vi "Gas_Release_Control.vi"(5 "Extra Commands":string, 6 "Density Ratio":string="Carrier 1 only", 7 "Strength (% by volume)":dbl format="%.3f", 8 "Stack flowrate (l/min)":dbl format="%.2f", 9 "Source Status":T2) -> (0 "error out":errorcluster, 1 "Flowrates (kg/min)":dbl[](array[numeric]) format="%.2f", 2 "Source Est Time (s)":dbl, 3 "Flowrates Achieved?":bool)   [LabVIEW 2013]
uses:
  ADAM Controls/Client_Source_Status.ctl
  ADAM Controls/Client_Source.ctl
  ADAM Controls/Channel_names.ctl
  ADAM Controls/Module_type_ADAM.ctl
  ADAM Controls/Calib_type_ADAM.ctl
  ADAM Controls/Channel_State.ctl
  ADAM Controls/Ch_description_ADAM.ctl
  ADAM Controls/Function_ADAM.ctl
  ADAM Controls/Address.ctl
  ADAM Controls/Update_scan_value.ctl
  Anemometry/Anemometry Sub Vis/Controls/In_Range.ctl
  Anemometry/Anemometry Sub Vis/Globals/Preference_global.vi
  Anemometry/Anemometry Sub Vis/Globals/Extra_Commands_Global.vi
panel:
  out "Error String":string
  out "Currently on":T1=enum."Get Source Clients"
  out "Status of other Clients":string[](array[string])
  out "Source already correct?":bool
  out "No Other Clients are Using Source?":bool
  out "Source Clients":string[](array[string])
  # "-Carrier 1 only\n-Carrier 2 only\n-Enter Ratio"
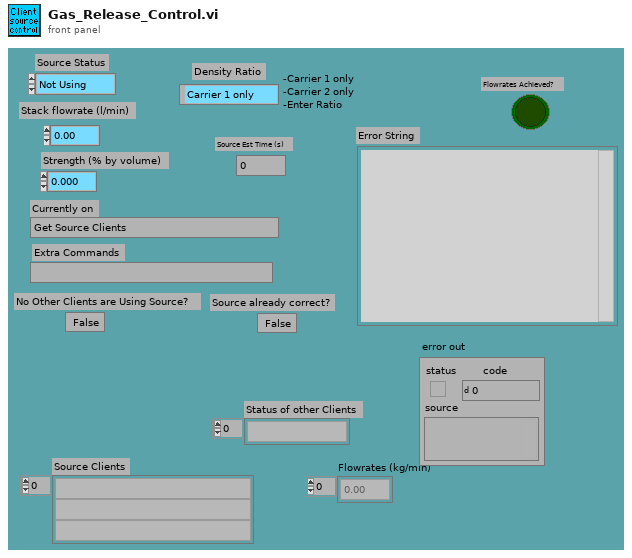
[diagram p1: front panel]
types:
  T1 = typedef "Client_Source.ctl" = enum16{"Start", "Get Source Clients", "Has this client liberty to control the source?", "Declare not using, other client already waiting", "Is the Source already correct?", "Declare waiting, other client is still using", "Control Hi-Tec", "Were the Hi-tecs able to achieve the flowrates?", "Declare source status", "Wait for source to Establish"}
  T2 = typedef "Client_Source_Status.ctl" = enum16{"Not Using", "Using", "Must Have"}
  T3 = typedef "Channel_names.ctl" = enum16{"Active Only", "Active + Off", "All Channels"}
  T4 = typedef "Ch_description_ADAM.ctl" = cluster{"Ch Name":string, "Type":T5, "Function":T6, "Ch State":T7, "Calibration type":T8, "A":dbl, "B":dbl, "C":dbl, "D":dbl, "Comments":string, "Address":T9, "String":string, "Duty":u16}
  T5 = typedef "Module_type_ADAM.ctl" = string
  T6 = typedef "Function_ADAM.ctl" = enum16{"Analogue Input", "Digital Input", "Event counter", "Event rate", "Analogue Output", "Digital Output", "Relay Output"}
  T7 = typedef "Channel_State.ctl" = enum16{"On", "Off", "Always On", "Always Off"}
  T8 = typedef "Calib_type_ADAM.ctl" = enum16{"Raw", "Bx + A", "Cx^2 + Bx + A", "Dx^3 + Cx^2 + Bx + A", "In Band", "Hi-Tec Q", "Hi-Tec M_dot", "Text"}
  T9 = typedef "Address.ctl" = cluster{"Main":i32, "Ch.":i32, "Sub":i32, "Port Name":string}
  T10 = typedef "Update_scan_value.ctl" = cluster{"Channel Name":string, "New Value":dbl}
  T11 = typedef "In_Range.ctl" = enum16{"%", "±", "% & ±"}
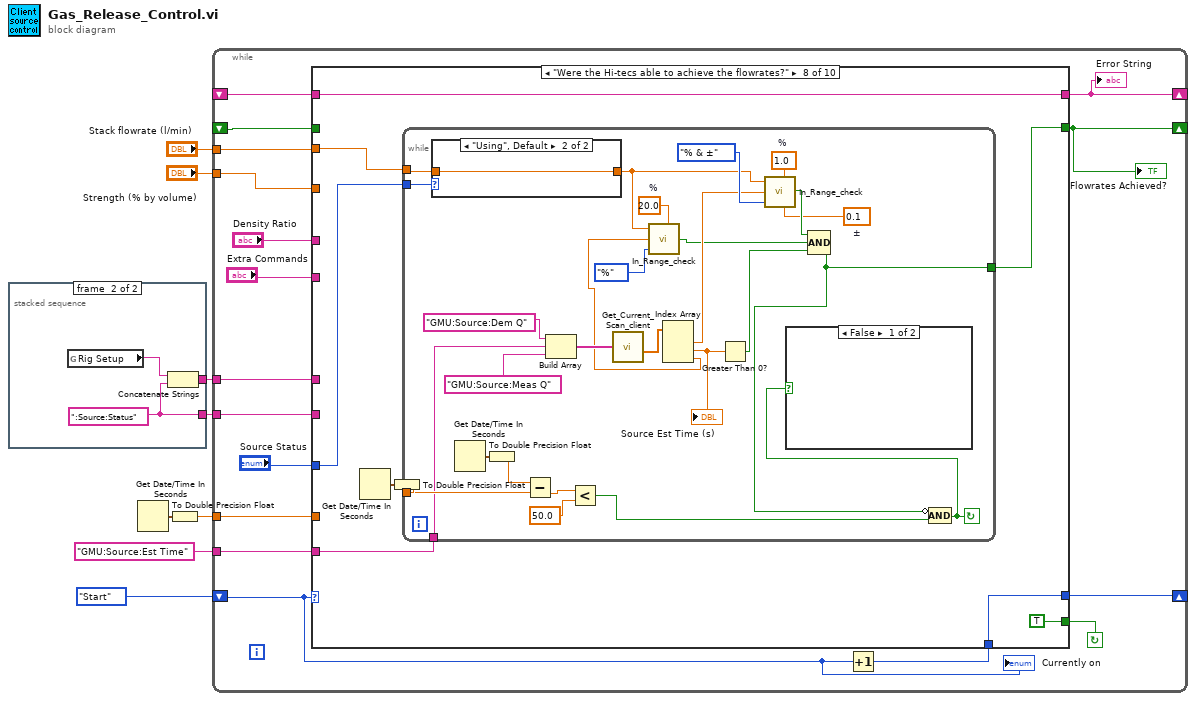
[diagram p0: block diagram]
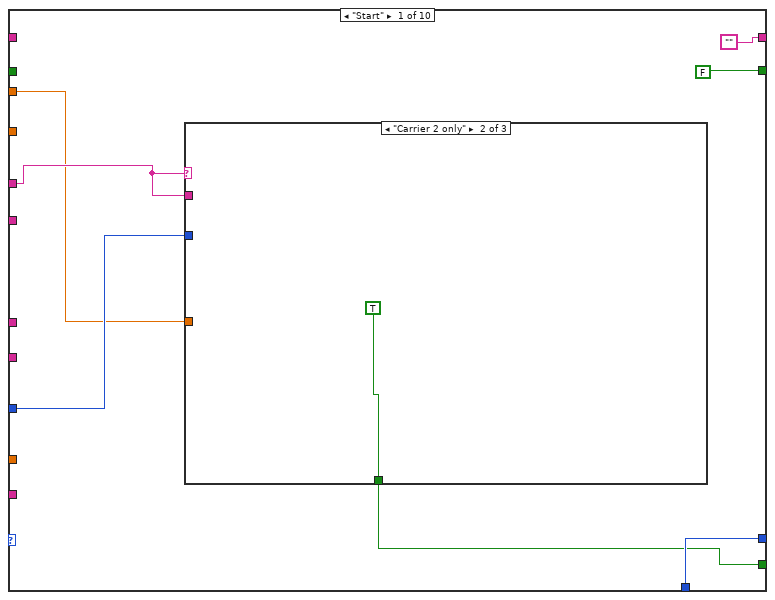
[diagram p2: hidden frame]
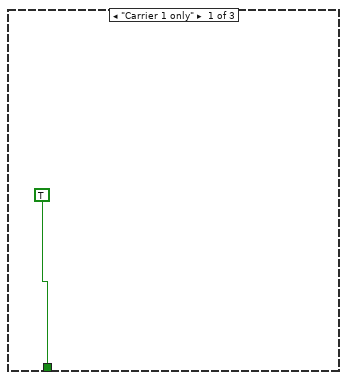
[diagram p3: hidden frame]
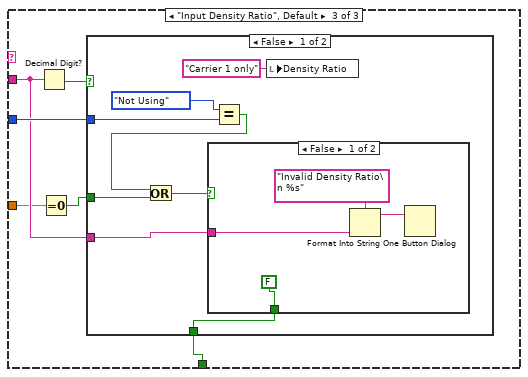
[diagram p4: hidden frame]
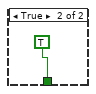
[diagram p5: hidden frame]
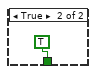
[diagram p6: hidden frame]
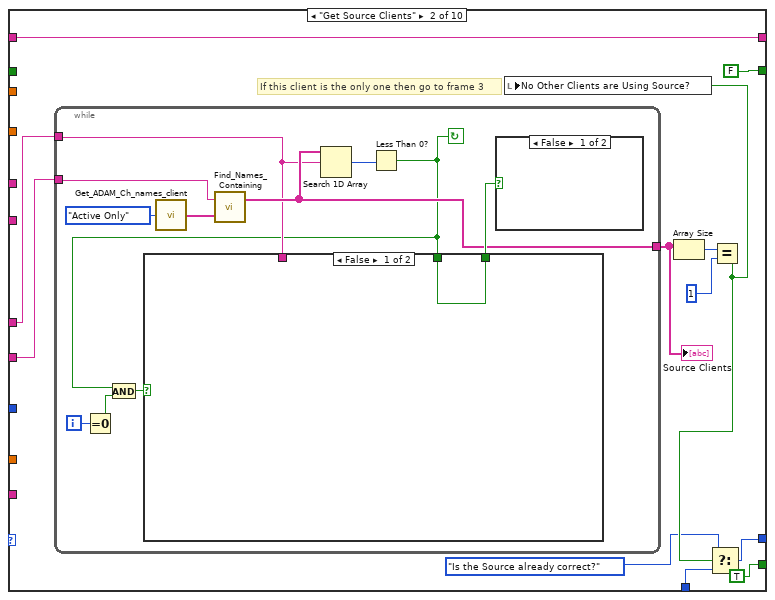
[diagram p7: hidden frame]
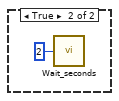
[diagram p8: hidden frame]
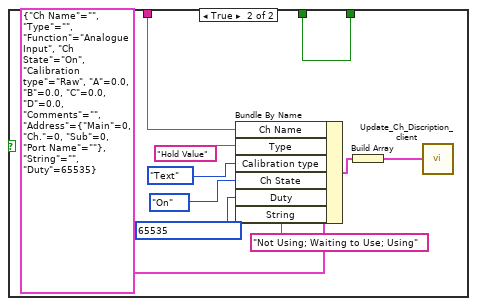
[diagram p9: hidden frame]
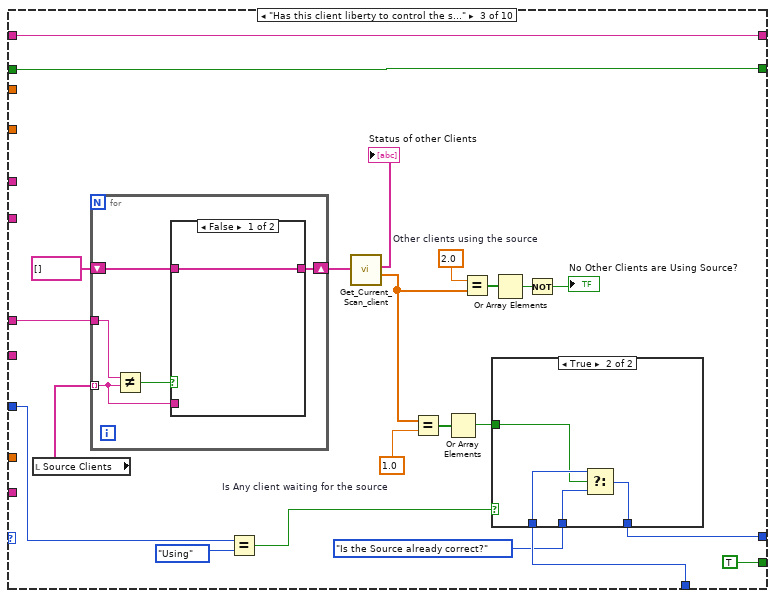
[diagram p10: hidden frame]
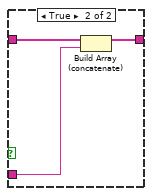
[diagram p12: hidden frame]
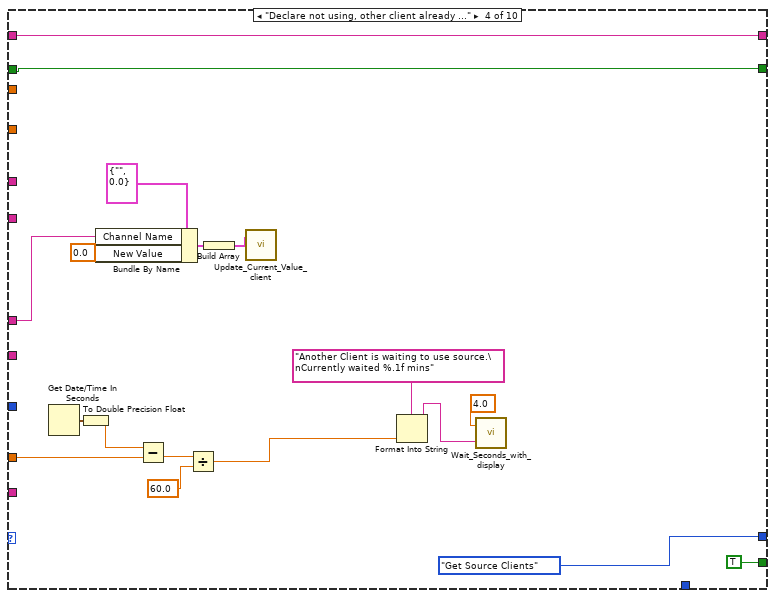
[diagram p13: hidden frame]
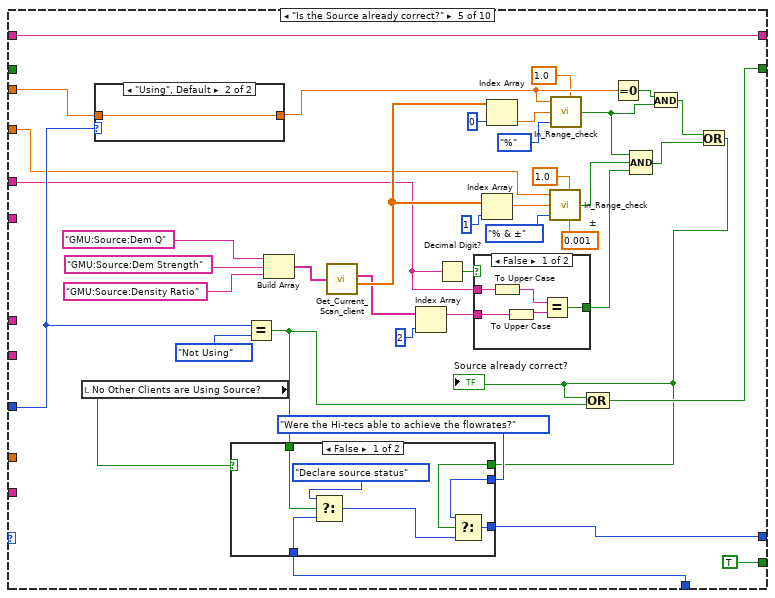
[diagram p14: hidden frame]
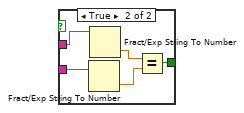
[diagram p15: hidden frame]
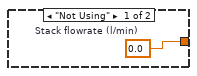
[diagram p16: hidden frame]
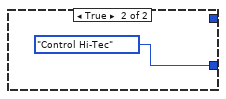
[diagram p17: hidden frame]
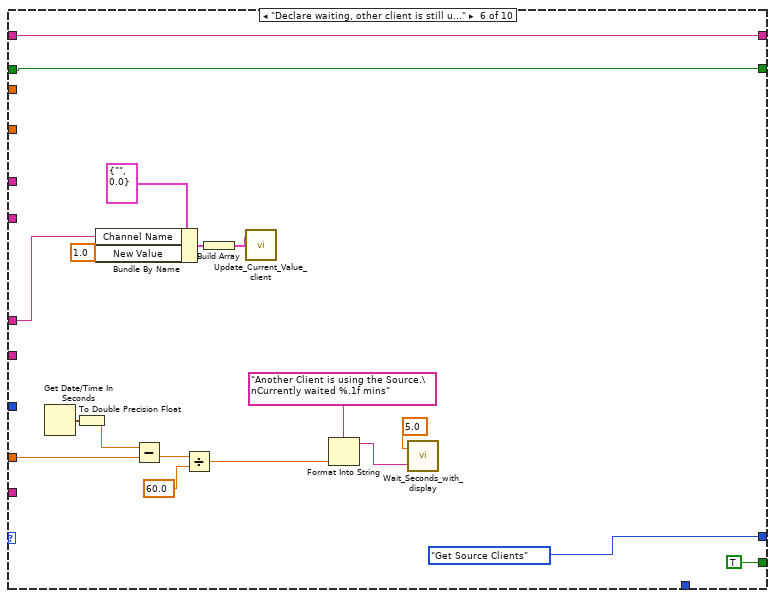
[diagram p18: hidden frame]
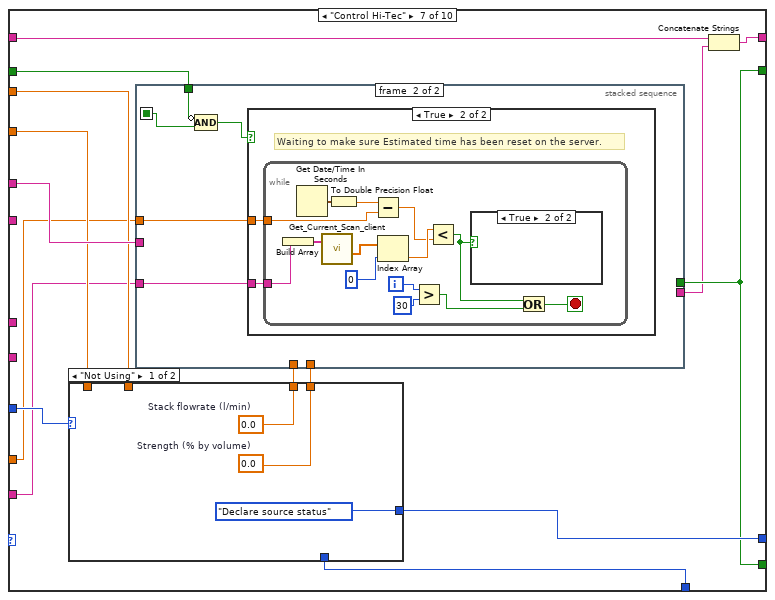
[diagram p19: hidden frame]
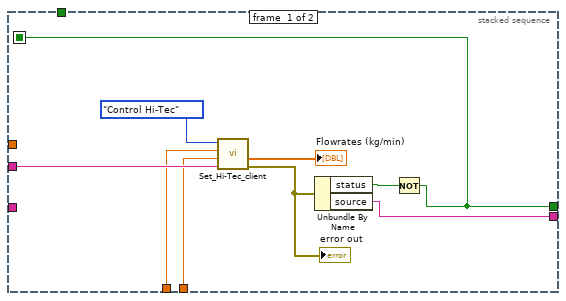
[diagram p20: hidden frame]
diagram:
  n1 = stacked-sequence {
    tunnel: [_ w11] -> w8
    tunnel: [_ w10] -> w7
    frame #0 {
      n2 = call "Run_EnFlo_Hub.vi"() -> ()  [unwired: 8 out]
    }
    frame #1 {
      w11 = ":Source:Status"
      n3 = global read "Preference_global.vi" "Rig Setup"() -> (w9:string)
      n4 = Concatenate Strings(w9, w11) -> (w10:string)
    }
  }
  n5 = Get Date/Time In Seconds() -> (seconds since 1Jan1904=w2:timestamp)
  n6 = To Double Precision Float(number=w2) -> (double precision float=w6:dbl)
  n7 = while {
    tunnel: w6 -> [w24]
    tunnel: w7 -> [w27]
    shift-left: Client_Source."Start" -> [w22]
    shift-right: [w23] -> _
    tunnel: w8 -> [w28]
    tunnel: "Stack flowrate (l/min)" -> [w18]
    tunnel: "Strength (% by volume)" -> [w17]
    shift-right: [w15] -> _
    shift-left: _ -> [w16]
    tunnel: "GMU:Source:Est Time" -> [w14]
    shift-right: [w12] -> _
    shift-left: _ -> [w13]
    stop <- w26 continue-if-true
    n8 = Increment(x=w22) -> (x+1=w25:T1)
    n9 = case shown="\"Were the Hi-tecs able to achieve the flowrates?\"" w22 {
      tunnel: w18 -> [w30 _ _ _ w178 _ w235 w281 _ w339]
      tunnel: w17 -> [_ _ _ _ w161 _ w233 _ _ _]
      tunnel: "Density Ratio" -> [w34 _ _ _ w153 _ w238 _ _ _]
      tunnel: w28 -> [_ w69 _ _ _ _ _ _ _ _]
      tunnel: [w35 w65 w107 Client_Source."Get Source Clients" w149 Client_Source."Get Source Clients" w232 w282 w323 w345] -> w23
      tunnel: w27 -> [_ w68 w114 w141 _ w218 _ _ w325 _]
      tunnel: [w33 TRUE TRUE TRUE TRUE TRUE w228 TRUE w317 FALSE] -> w26
      tunnel: w25 -> [w35 w64 w109 _ w179 _ w231 w282 w323 w345]
      tunnel: w24 -> [_ _ _ w139 _ w213 w229 _ _ _]
      tunnel: "Source Status" -> [w32 _ w98 _ w170 _ w237 w280 w324 w344]
      tunnel: "Extra Commands" -> [_ _ _ _ _ _ _ _ _ w342]
      tunnel: [FALSE FALSE w94 w131 w151 w208 w228 w279 w318 w340] -> w15
      tunnel: w16 -> [_ _ w94 w131 _ w208 w227 _ w318 w340]
      tunnel: w14 -> [_ _ _ _ _ _ w230 w277 _ _]
      tunnel: w13 -> [_ w58 w93 w129 w147 w206 w225 w276 w316 w338]
      tunnel: ["" w58 w93 w129 w147 w206 w226 w276 w315 w338] -> w12
      frame "Start" {
        n10 = case shown="\"Carrier 2 only\"" w34 {
          tunnel: w34 -> [_ _ w40]
          tunnel: [TRUE TRUE w41] -> w33
          tunnel: w32 -> [_ _ w42]
          tunnel: w30 -> [_ _ w39]
          frame "Carrier 1 only" {
            (unwired) TRUE
            (unwired) 0.0 ("Qc2")
          }
          frame "Carrier 2 only" {
            (unwired) TRUE
            (unwired) 0.0 ("Qc1")
          }
          frame "Input Density Ratio", Default {
            n11 = Decimal Digit?(1:w40) -> (0:w43:bool)
            n12 = Equal To 0?(x=w39) -> (x = 0?=w38:bool)
            n13 = case shown="False" w43 {
              tunnel: w42 -> [w50 _]
              tunnel: [w49 TRUE] -> w41
              tunnel: w40 -> [w48 _]
              tunnel: w38 -> [w45 _]
              frame False {
                n14 = Equal?(x=Client_Source_Status."Not Using" ("Source Status"), y=w50) -> (x = y?=w46:bool)
                n15 = Or(x=w46, y=w45) -> (x .or. y?=w44:bool)
                n16 = case shown="False" w44 {
                  tunnel: [FALSE TRUE] -> w49
                  tunnel: w48 -> [w55 _]
                  frame False {
                    n17 = Format Into String(format string="Invalid Density Ratio\n %s", w55) -> (resulting string=w53:string)  [unwired: 2 in, 1 out]
                    n18 = One Button Dialog(message=w53) -> ()  [unwired: 2 out]
                  }
                  frame True {
                  }
                }
                n19 = local write "Density Ratio"("Carrier 1 only" ("Density Ratio")) -> ()
              }
              frame True {
              }
            }
          }
        }
      }
      frame "Get Source Clients" {
        # "If this client is the only one then go to frame 3"
        n20 = while {
          tunnel: [w73] -> w62
          tunnel: w68 -> [w72]
          tunnel: w69 -> [w80]
          i -> [w77]
          stop <- w70 continue-if-true
          n21 = Equal To 0?(x=w77) -> (x = 0?=w76:bool)
          n22 = call "Get_ADAM_Ch_names_client.vi"("Channel names set"=Channel_names."Active Only") -> ("Ch names"=w78:string[])
          n23 = call "Find_Names_Containing.vi"("Ch names"=w78, "String to match"=w80) -> ("Matched Names"=w73:string[])  [unwired: 1 out]
          n24 = Search 1D Array(1D array=w73, element=w72) -> (index of element=w71:i32)  [unwired: 1 out]
          n25 = Less Than 0?(x=w71) -> (x < 0?=w70:bool)
          n26 = And(x=w70, y=w76) -> (x .and. y?=w75:bool)
          n27 = case shown="False" w75 {
            tunnel: w72 -> [_ w89]
            tunnel: [w82 w85] -> w74
            tunnel: w70 -> [w82 w85]
            frame False {
            }
            frame True {
              n28 = Bundle By Name(cluster=T4 {"Ch Name"="", "Type"="", "Function"=enum."Analogue Input", "Ch State"=enum."On", "Calibration type"=enum."Raw", "A"=0.0, "B"=0.0, "C"=0.0, "D"=0.0, "Comments"="", "Address"={"Main"=0, "Ch."=0, "Sub"=0, "Port Name"=""}, "String"="", "Duty"=65535} ("Ch Discription"), "Ch Name"=w89, "Type"=T5 "Hold Value", "Calibration type"=Calib_type_ADAM."Text", "Ch State"=Channel_State."On", "Duty"=u16 65535 ("Bundle Element"), "String"="Not Using; Waiting to Use; Using") -> (w87:T4)
              n29 = Build Array(w87) -> (w86:T4[])
              n30 = call "Update_Ch_Discription_client.vi"("Channels to update In"=w86) -> ()  [unwired: 1 out]
            }
          }
          n31 = case shown="False" w74 {
            frame False {
            }
            frame True {
              n32 = call "Wait_seconds.vi"("Seconds to wait"=u32 2) -> ()
            }
          }
        }
        "Source Clients" <- w62
        n33 = Array Size(array=w62) -> (size(s)=w67:i32)
        n34 = Equal?(x=w67, y=1) -> (x = y?=w61:bool)
        n35 = local write "No Other Clients are Using Source?"(w61) -> ()
        n36 = Select(t=Client_Source."Is the Source already correct?", s=w61, f=w64) -> (s? t:f=w65:T1)
      }
      frame "Has this client liberty to control the source?" {
        w106 = 2.0  # Other clients using the source
        w112 = 1.0  # Is Any client waiting for the source
        n37 = local read "Source Clients"() -> (w108:string[])
        n38 = for {
          tunnel: w108 -> [w120] mode=indexing
          tunnel: w114 -> [w124]
          shift-right: [w121] -> w104
          shift-left: string[] [] -> [w122]
          n39 = Not Equal?(x=w124, y=w120) -> (x != y?=w123:bool)
          n40 = case shown="False" w123 {
            tunnel: w122 -> [w125 w128]
            tunnel: [w125 w127] -> w121
            tunnel: w120 -> [_ w126]
            frame False {
            }
            frame True {
              n41 = Build Array (concatenate)(w128, w126) -> (w127:string[])
            }
          }
        }
        n42 = Equal?(x=w98, y=Client_Source_Status."Using" ("Source Status")) -> (x = y?=w97:bool)
        n43 = call "Get_Current_Scan_client.vi"("ADAM Ch Names"=w104) -> ("String values"=→"Status of other Clients":string[], "Numerical Values"=w101:dbl[])  [unwired: 2 out]
        n44 = Equal?(x=w101, y=w112) -> (x = y?=w111:bool[])
        n45 = Or Array Elements(Boolean array=w111) -> (logical OR=w102:bool)
        n46 = Equal?(x=w106, y=w101) -> (x = y?=w105:bool[])
        n47 = case shown="True" w97 {
          tunnel: w109 -> [_ w119]
          tunnel: [w115 w118] -> w107
          tunnel: w102 -> [_ w117]
          tunnel: Client_Source."Is the Source already correct?" -> [w115 w116]
          frame False {
          }
          frame True {
            n48 = Select(t=w119, s=w117, f=w116) -> (s? t:f=w118:T1)
          }
        }
        n49 = Or Array Elements(Boolean array=w105) -> (logical OR=w100:bool)
        n50 = Not(x=w100) -> (.not. x?=→"No Other Clients are Using Source?":bool)
      }
      frame "Declare not using, other client already waiting" {
        n51 = Get Date/Time In Seconds() -> (seconds since 1Jan1904=w130:timestamp)
        n52 = To Double Precision Float(number=w130) -> (double precision float=w140:dbl)
        n53 = Bundle By Name(cluster=T10 {"Channel Name"="", "New Value"=0.0} ("Update Scan Value Cluster"), "Channel Name"=w141, "New Value"=0.0 ("Bundle Element")) -> (w144:T10)
        n54 = Subtract(x=w140, y=w139) -> (x-y=w138:dbl)
        n55 = Divide(x=w138, y=60.0) -> (x/y=w132:dbl)
        n56 = Build Array(w144) -> (w143:T10[])
        n57 = call "Update_Current_Value_client.vi"("Update array in"=w143) -> ()  [unwired: 1 in]
        n58 = Format Into String(format string="Another Client is waiting to use source.\nCurrently waited %.1f mins" ("Format String"), w132) -> (resulting string=w135:string)  [unwired: 2 in, 1 out]
        n59 = call "Wait_Seconds_with_display.vi"("Message"=w135, "Seconds to wait"=4.0) -> ()  [unwired: 2 out]
      }
      frame "Is the Source already correct?" {
        w158 = 0.001  # ±
        n60 = local read "No Other Clients are Using Source?"() -> (w180:bool)
        n61 = case shown="\"Using\", Default" w170 {
          tunnel: [w196 w197] -> w168
          tunnel: w178 -> [_ w197]
          frame "Not Using" {
            w196 = 0.0  # Stack flowrate (l/min)
          }
          frame "Using", Default {
          }
        }
        n62 = Equal?(x=w170, y=Client_Source_Status."Not Using" ("Source Status")) -> (x = y?=w169:bool)
        n63 = Build Array("GMU:Source:Dem Q", "GMU:Source:Dem Strength", "GMU:Source:Density Ratio") -> (w182:string[])
        n64 = call "Get_Current_Scan_client.vi"("ADAM Ch Names"=w182) -> ("String values"=w155:string[], "Numerical Values"=w175:dbl[])  [unwired: 2 out]
        n65 = Index Array(array=w155, index=2 ("Index")) -> (element=w154:string)
        n66 = Decimal Digit?(1:w153) -> (0:w157:bool)
        n67 = case shown="False" w157 {
          tunnel: [w189 w192] -> w152
          tunnel: w153 -> [w188 w194]
          tunnel: w154 -> [w187 w195]
          frame False {
            n68 = To Upper Case(1:w188) -> (0:w190:string)
            n69 = To Upper Case(1:w187) -> (0:w186:string)
            n70 = Equal?(x=w190, y=w186) -> (x = y?=w189:bool)
          }
          frame True {
            n71 = Fract/Exp String To Number(string=w195) -> (number=w191:dbl)  [unwired: 4 out]
            n72 = Fract/Exp String To Number(string=w194) -> (number=w193:dbl)  [unwired: 4 out]
            n73 = Equal?(x=w193, y=w191) -> (x = y?=w192:bool)
          }
        }
        n74 = Index Array(array=w175, index=1 ("Index")) -> (element=w160:dbl)
        n75 = Index Array(array=w175, index=0 ("Index")) -> (element=w167:dbl)
        n76 = call "In_Range_check.vi"("±"=w158, "%"=1.0, "Mode"=In_Range."% & ±", "Value"=w160, "Setpoint"=w161) -> ("In Range"=w159:bool)  [unwired: 2 out]
        n77 = call "In_Range_check.vi"("%"=1.0, "Mode"=In_Range."%", "Value"=w167, "Setpoint"=w168) -> ("In Range"=w166:bool)  [unwired: 1 in, 2 out]
        n78 = Equal To 0?(x=w168) -> (x = 0?=w174:bool)
        n79 = Compound Arithmetic op=AND(w166, w159, w152) -> (w172:bool)
        n80 = And(x=w174, y=w166) -> (x .and. y?=w173:bool)
        n81 = Or(x=w173, y=w172) -> (x .or. y?=w148:bool)
        "Source already correct?" <- w148
        n82 = case shown="False" w180 {
          tunnel: w179 -> [w204 _]
          tunnel: w169 -> [w203 _]
          tunnel: w148 -> [w201 _]
          tunnel: Client_Source."Were the Hi-tecs able to achieve the flowrates?" -> [w199 _]
          tunnel: [w198 Client_Source."Control Hi-Tec"] -> w149
          frame False {
            n83 = Select(t=Client_Source."Declare source status", s=w203, f=w204) -> (s? t:f=w200:T1)
            n84 = Select(t=w199, s=w201, f=w200) -> (s? t:f=w198:T1)
          }
          frame True {
          }
        }
        n85 = Compound Arithmetic op=OR(w148, w169) -> (w151:bool)
      }
      frame "Declare waiting, other client is still using" {
        n86 = Get Date/Time In Seconds() -> (seconds since 1Jan1904=w207:timestamp)
        n87 = To Double Precision Float(number=w207) -> (double precision float=w216:dbl)
        n88 = Bundle By Name(cluster=T10 {"Channel Name"="", "New Value"=0.0} ("Update Scan Value Cluster"), "Channel Name"=w218, "New Value"=1.0 ("Bundle Element")) -> (w221:T10)
        n89 = Subtract(x=w216, y=w213) -> (x-y=w215:dbl)
        n90 = Divide(x=w215, y=60.0) -> (x/y=w209:dbl)
        n91 = Build Array(w221) -> (w220:T10[])
        n92 = call "Update_Current_Value_client.vi"("Update array in"=w220) -> ()  [unwired: 1 in]
        n93 = Format Into String(format string="Another Client is using the Source.\nCurrently waited %.1f mins" ("Format String"), w209) -> (resulting string=w212:string)  [unwired: 2 in, 1 out]
        n94 = call "Wait_Seconds_with_display.vi"("Message"=w212, "Seconds to wait"=5.0) -> ()  [unwired: 2 out]
      }
      frame "Control Hi-Tec" {
        n95 = case shown="\"Not Using\"" w237 {
          tunnel: [w272 w275] -> w236
          tunnel: w235 -> [_ w275]
          tunnel: [w271 w274] -> w234
          tunnel: w233 -> [_ w274]
          tunnel: [Client_Source."Declare source status" w273] -> w232
          tunnel: w231 -> [_ w273]
          frame "Not Using" {
            w271 = 0.0  # Strength (% by volume)
            w272 = 0.0  # Stack flowrate (l/min)
          }
          frame "Using", Default {
          }
        }
        n96 = stacked-sequence {
          seq-local: [w240 _] -> [_ w250]
          tunnel: w238 -> [w246 _]
          tunnel: w236 -> [w244 _]
          tunnel: w234 -> [w243 _]
          tunnel: w230 -> [_ w252]
          tunnel: w229 -> [_ w251]
          tunnel: [w240 _] -> w228
          tunnel: w227 -> [_ w249]
          tunnel: [w239 _] -> w224
          frame #0 {
            n97 = call "Set_Hi-Tec_client.vi"("Density Ratio"=w246, "Strength (% by volume)"=w243, "Stack flowrate (l/min)"=w244, "Mode"=enum16{"Control Hi-Tec", "Check Hi-Tec Demands"}."Control Hi-Tec") -> ("error out"=w242:errorcluster, "Flowrates (kg/min)"=→"Flowrates (kg/min)":dbl[])  [unwired: 1 in, 3 out]
            "error out" <- w242
            n98 = Unbundle By Name(w242) -> ("status"=w241:bool, "source"=w239:string)
            n99 = Not(x=w241) -> (.not. x?=w240:bool)
          }
          frame #1 {
            n100 = Compound Arithmetic op=AND(invert w249, w250) -> (w248:bool)
            n101 = case shown="True" w248 {
              tunnel: w252 -> [_ w254]
              tunnel: w251 -> [_ w253]
              frame False {
              }
              frame True {
                # "Waiting to make sure Estimated time has been reset on the server."
                n102 = while {
                  tunnel: w254 -> [w267]
                  tunnel: w253 -> [w262]
                  i -> [w259]
                  stop <- w255 stop-if-true
                  n103 = Build Array(w267) -> (w268:string[])
                  n104 = Get Date/Time In Seconds() -> (seconds since 1Jan1904=w264:timestamp)
                  n105 = call "Get_Current_Scan_client.vi"("ADAM Ch Names"=w268) -> ("Numerical Values"=w266:dbl[])  [unwired: 3 out]
                  n106 = To Double Precision Float(number=w264) -> (double precision float=w263:dbl)
                  n107 = Subtract(x=w263, y=w262) -> (x-y=w260:dbl)
                  n108 = Index Array(array=w266, index=0) -> (element=w261:dbl)
                  n109 = Greater?(x=w259, y=30) -> (0:w256:bool)
                  n110 = Less?(x=w261, y=w260) -> (x < y?=w257:bool)
                  n111 = case shown="True" w257 {
                    frame False {
                      n112 = Wait (ms)(milliseconds to wait=u32 1000) -> ()  [unwired: 1 out]
                    }
                    frame True {
                    }
                  }
                  n113 = Or(x=w257, y=w256) -> (x .or. y?=w255:bool)
                }
              }
            }
          }
        }
        n114 = Concatenate Strings(w225, w224) -> (w226:string)
      }
      frame "Were the Hi-tecs able to achieve the flowrates?" {
        n115 = Get Date/Time In Seconds() -> (seconds since 1Jan1904=w278:timestamp)
        n116 = To Double Precision Float(number=w278) -> (double precision float=w283:dbl)
        n117 = while {
          tunnel: w280 -> [w300]
          tunnel: w281 -> [w299]
          tunnel: w283 -> [w309]
          tunnel: [w297] -> w279
          tunnel: w277 -> [w295]
          stop <- w306 continue-if-true
          w285 = 20.0  # %
          w298 = 0.1  # ±
          w304 = 1.0  # %
          n118 = case shown="\"Using\", Default" w300 {
            tunnel: [w312 w313] -> w287
            tunnel: w299 -> [_ w313]
            frame "Not Using" {
              w312 = 0.0  # Stack flowrate (l/min)
            }
            frame "Using", Default {
            }
          }
          n119 = Get Date/Time In Seconds() -> (seconds since 1Jan1904=w296:timestamp)
          n120 = To Double Precision Float(number=w296) -> (double precision float=w310:dbl)
          n121 = Subtract(x=w310, y=w309) -> (x-y=w286:dbl)
          n122 = Build Array("GMU:Source:Dem Q", w295, "GMU:Source:Meas Q") -> (w311:string[])
          n123 = Less?(x=w286, y=50.0) -> (x < y?=w307:bool)
          n124 = call "Get_Current_Scan_client.vi"("ADAM Ch Names"=w311) -> ("Numerical Values"=w302:dbl[])  [unwired: 3 out]
          n125 = Index Array(array=w302) -> (element #1=w290:dbl, element #2=w293:dbl, element #3=w291:dbl)  [unwired: 3 in]
          "Source Est Time (s)" <- w293
          n126 = call "In_Range_check.vi"("%"=w285, "Mode"=In_Range."%", "Value"=w291, "Setpoint"=w287) -> ("In Range"=w288:bool)  [unwired: 1 in, 2 out]
          n127 = Greater Than 0?(x=w293) -> (x > 0?=w289:bool)
          n128 = call "In_Range_check.vi"("±"=w298, "%"=w304, "Mode"=In_Range."% & ±", "Value"=w290, "Setpoint"=w287) -> ("In Range"=w301:bool)  [unwired: 2 out]
          n129 = Compound Arithmetic op=AND(w301, w288, w289) -> (w297:bool)
          n130 = Compound Arithmetic op=AND(invert w297, w307) -> (w306:bool)
          n131 = case shown="False" w306 {
            frame False {
            }
            frame True {
              n132 = Wait (ms)(milliseconds to wait=u32 1000) -> ()  [unwired: 1 out]
            }
          }
        }
      }
      frame "Declare source status" {
        n133 = case shown="False" w318 {
          tunnel: w324 -> [_ w334]
          tunnel: [0.0 w333] -> w319
          tunnel: [FALSE TRUE] -> w317
          tunnel: w316 -> [w327 w331]
          tunnel: [w326 w331] -> w315
          frame False {
            n134 = Concatenate Strings(w327, "Requested Flowrate has not been acheived.\n" ("Error String")) -> (w326:string)
          }
          frame True {
            n135 = case shown="\"Using\"" w334 {
              tunnel: [0.0 2.0 2.0] -> w333
              frame "Not Using" {
              }
              frame "Using" {
              }
              frame "Must Have" {
              }
            }
          }
        }
        n136 = Bundle By Name(cluster=T10 {"Channel Name"="", "New Value"=0.0} ("Update Scan Value Cluster"), "Channel Name"=w325, "New Value"=w319) -> (w321:T10)
        n137 = Build Array(w321) -> (w320:T10[])
        n138 = call "Update_Current_Value_client.vi"("Update array in"=w320) -> ()  [unwired: 1 in]
      }
      frame "Wait for source to Establish" {
        n139 = Not Equal?(x=Client_Source_Status."Not Using" ("Source Status"), y=w344) -> (x != y?=w341:bool)
        n140 = case shown="True" w341 {
          tunnel: w342 -> [_ w363]
          tunnel: w339 -> [_ w352]
          frame False {
          }
          frame True {
            n141 = global read "Extra_Commands_Global.vi" "Establish Exp Conditions (s)"() -> (w364:string)
            n142 = global read "Preference_global.vi" "Default Source Establishment Time (s)"() -> (w355:dbl)
            n143 = Equal To 0?(x=w352) -> (x = 0?=w350:bool)
            n144 = Divide(x=100.0, y=w352) -> (x/y=w349:dbl)
            n145 = local read "Source Est Time (s)"() -> (w356:dbl)
            n146 = Not A Number/Path/Refnum?(number/path/refnum=w356) -> (NaN/Path/Refnum?=w360:bool)
            n147 = call "Extra_Commands.vi"("String to Search"=w363, "Command"=w364) -> ("Numeric Value"=w357:dbl, "Command Found"=w358:bool)  [unwired: 1 in, 3 out]
            n148 = Select(t=w357, s=w358, f=w355) -> (s? t:f=w354:dbl)
            n149 = Select(t=0.0, s=w350, f=w349) -> (s? t:f=w347:dbl)
            n150 = Add(x=w347, y=w354) -> (x+y=w353:dbl)
            n151 = Subtract(x=w353, y=w356) -> (x-y=w359:dbl)
            n152 = Greater Than 0?(x=w359) -> (x > 0?=w362:bool)
            n153 = Or(x=w362, y=w360) -> (x .or. y?=w361:bool)
            n154 = case shown="True" w361 {
              tunnel: w360 -> [_ w368]
              tunnel: w353 -> [_ w367]
              tunnel: w359 -> [_ w366]
              frame False {
              }
              frame True {
                n155 = Select(t=w367, s=w368, f=w366) -> (s? t:f=w365:dbl)
                n156 = call "Wait_Seconds_with_display.vi"("Message"="Establishing Source", "Seconds to wait"=w365) -> ()  [unwired: 2 out]
              }
            }
          }
        }
      }
    }
    "Flowrates Achieved?" <- w15
    "Error String" <- w12
    "Currently on" <- w22
  }
